vi "Write Datagram to Port.vi"(4 "destination address":u32, 6 "destination port":u16, 8 "error in (no error)":errorcluster, 9 "timeout ms (25000)":i32=25000 format="%d ms", 10 "data":string, 11 "UDP Transceiver in":refnum<class "UDP Transceiver.lvclass">) -> (0 "error out":errorcluster, 1 "timed out?":bool, 3 "UDP Transceiver out":refnum<class "UDP Transceiver.lvclass">)   [LabVIEW 2017, in "UDP.lvlib" / "UDP Transceiver.lvclass"]
uses:
  UDP Transceiver.lvclass
  UDP Transceiver.lvclass/UDP Transceiver.ctl
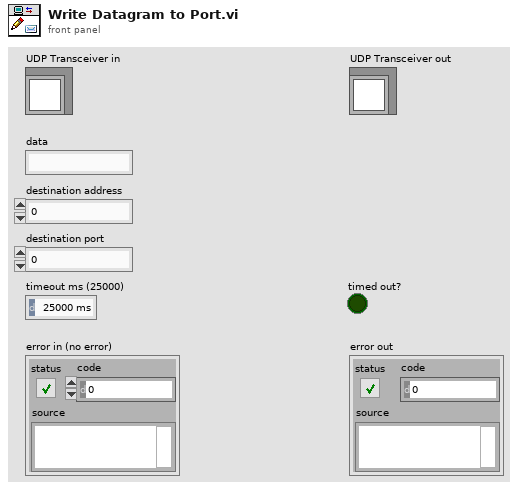
[diagram p1: front panel]
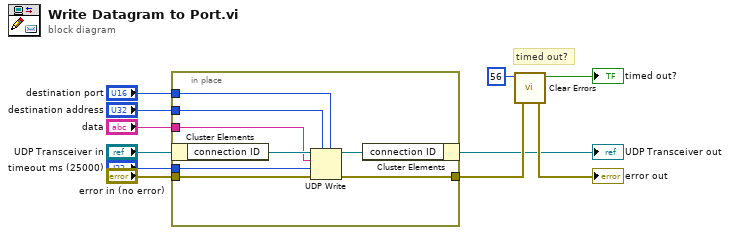
[diagram p0: block diagram]
diagram:
  # "timed out?"
  n1 = in-place {
    in-place-border: "error in (no error)" -> [w19]
    in-place-border: [w18] -> w10
    in-place-border: "timeout ms (25000)" -> [w16]
    in-place-border: "data" -> [w14]
    in-place-border: "destination address" -> [w13]
    in-place-border: "destination port" -> [w12]
    n2 = in-place-cluster #1("UDP Transceiver in") -> ("connection ID"=w17:refnum<k16>)
    n3 = UDP Write(address=w13, port or service name=w12, connection ID=w17, data in=w14, 8:w19, 9:w16) -> (error out=w18:errorcluster, 3:w15:refnum<k16>)
    n4 = in-place-cluster #1("connection ID"=w15) -> (→"UDP Transceiver out":refnum<class "UDP Transceiver.lvclass">)
  }
  n5 = call <vilib>:"Clear Errors.vi"("error in (no error)"=w10, "specific error code to clear (0: all)"=56) -> ("error out"=→"error out":errorcluster, "specific error cleared?"=→"timed out?":bool)  [unwired: 4 in]
